vi "fgv_hw-err.vi"(7 "cmd":enum16{"ini", "read", "write"}(ring), 11 "HW check":T1) -> (3 "HW check out":T1)   [LabVIEW 2019]
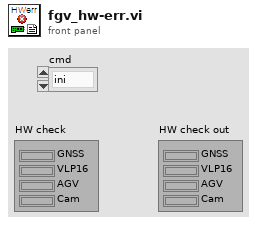
[diagram p1: front panel]
types:
  T1 = cluster{"GNSS":u16, "VLP16":u16, "AGV":u16, "Cam":u16}
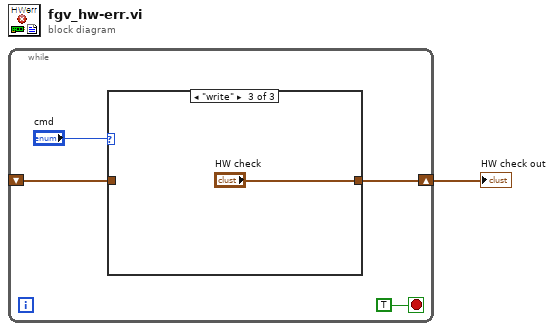
[diagram p0: block diagram]
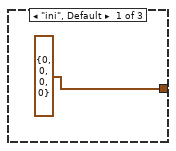
[diagram p2: hidden frame]
diagram:
  n1 = while {
    shift-right: [w3] -> w1
    shift-left: _ -> [w2]
    stop <- TRUE stop-if-true
    n2 = case shown="\"write\"" "cmd" {
      tunnel: [T1 {"GNSS"=0, "VLP16"=0, "AGV"=0, "Cam"=0} ("HW ceck 2") w7 "HW check"] -> w3
      tunnel: w2 -> [_ w7 _]
      frame "ini", Default {
      }
      frame "read" {
      }
      frame "write" {
      }
    }
  }
  "HW check out" <- w1
